vi "InstalMultiplePackages.vi"(8 "Error In":errorcluster, 9 "Include Recommended?":bool, 10 "Version":string, 11 "Package Name":string) -> (0 "Error Out":errorcluster, 3 "Installed Version":string)   [LabVIEW 2019]
uses:
  <vilib>/National Instruments/NIPM API (Beta)/NIPM_API.lvlib
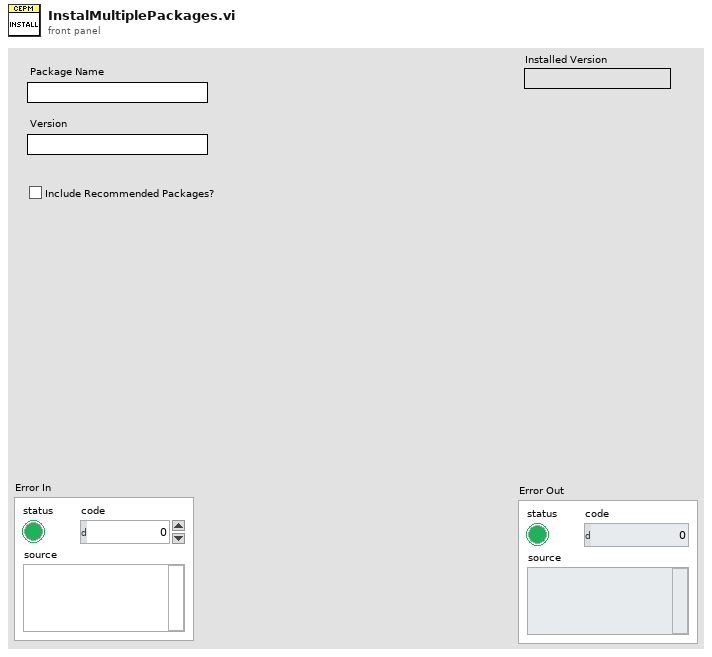
[diagram p1: front panel]
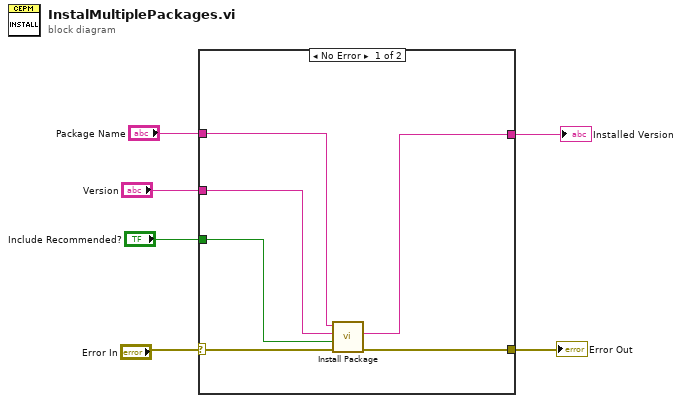
[diagram p0: block diagram]
diagram:
  n1 = case shown="No Error" "Error In" {
    selector: "Error In" -> [w12 w13]
    tunnel: [w11 w13] -> w5
    tunnel: "Package Name" -> [w10 _]
    tunnel: "Version" -> [w9 _]
    tunnel: [w8 _] -> w2
    tunnel: "Include Recommended?" -> [w7 _]
    frame No Error {
      n2 = call <vilib>:"Install Package.vi"("error in"=w12, "include recommended packages? (F)"=w7, "version"=w9, "package name"=w10) -> ("error out"=w11:errorcluster, "installed version"=w8:string)  [unwired: 5 in, 1 out]
    }
    frame Error {
    }
  }
  "Error Out" <- w5
  "Installed Version" <- w2
